vi "ReadTDMSFileFromHBM&Correct.vi"(4 "error in (no error)":errorcluster, 6 "file path":path) -> (0 "sortie d'erreur":errorcluster, 2 "HBMWaveformsOut":waveform(dbl)[](graph))   [LabVIEW 2017]
panel:
  out "Graphe":waveform(dbl)[](graph)
  out "iteraFinal":i32
  out "TabNomFinal":string[](array[string])
  out "ChannelNames 2":string[](array[string])
  out "size(s) 3":i32
  out "WaveformComputational":waveform(dbl)[](graph)
  out "ChannelUnit 2":string[](array[string])
  out "size(s) 2":i32
  out "Unit":string
  out "Name":string
  out "ChannelUnit":string[](array[string])
  out "ChannelNames":string[](array[string])
  out "Waveform Graph 2":waveform(dbl)(graph)
  out "WaveformHardware":waveform(dbl)[](graph)
  out "size(s)":i32
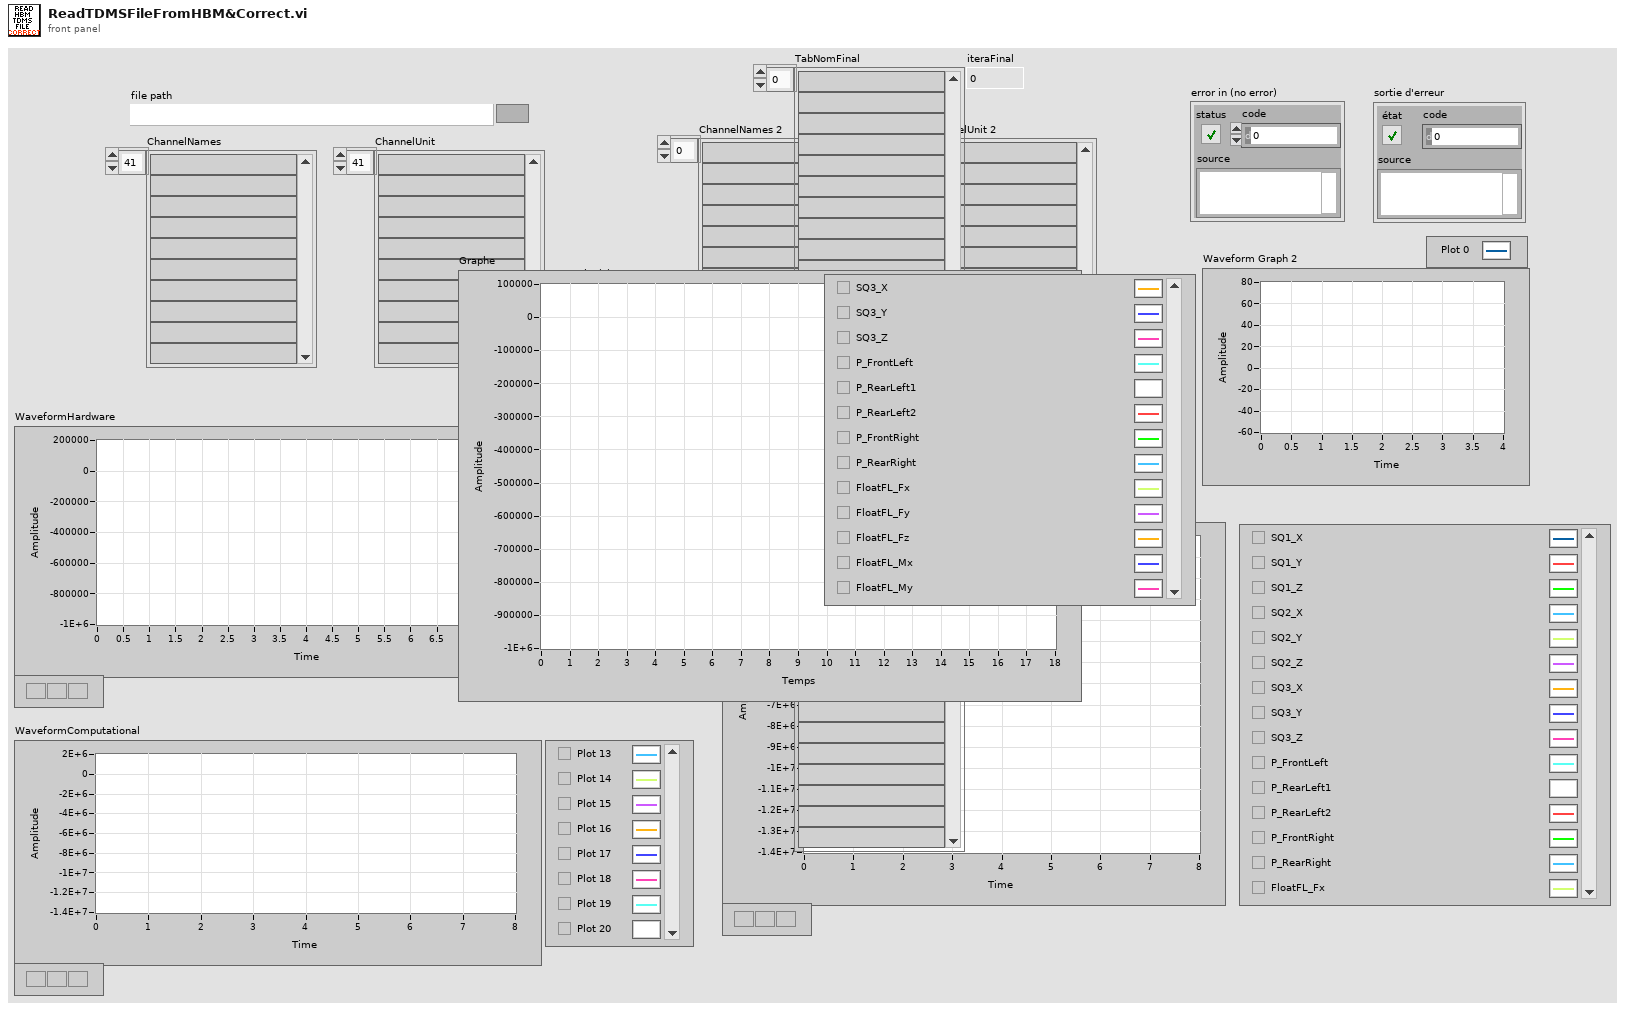
[diagram p1: front panel]
types:
  T1 = enum16{"open", "open or create", "create or replace", "create", "open (read-only)"}
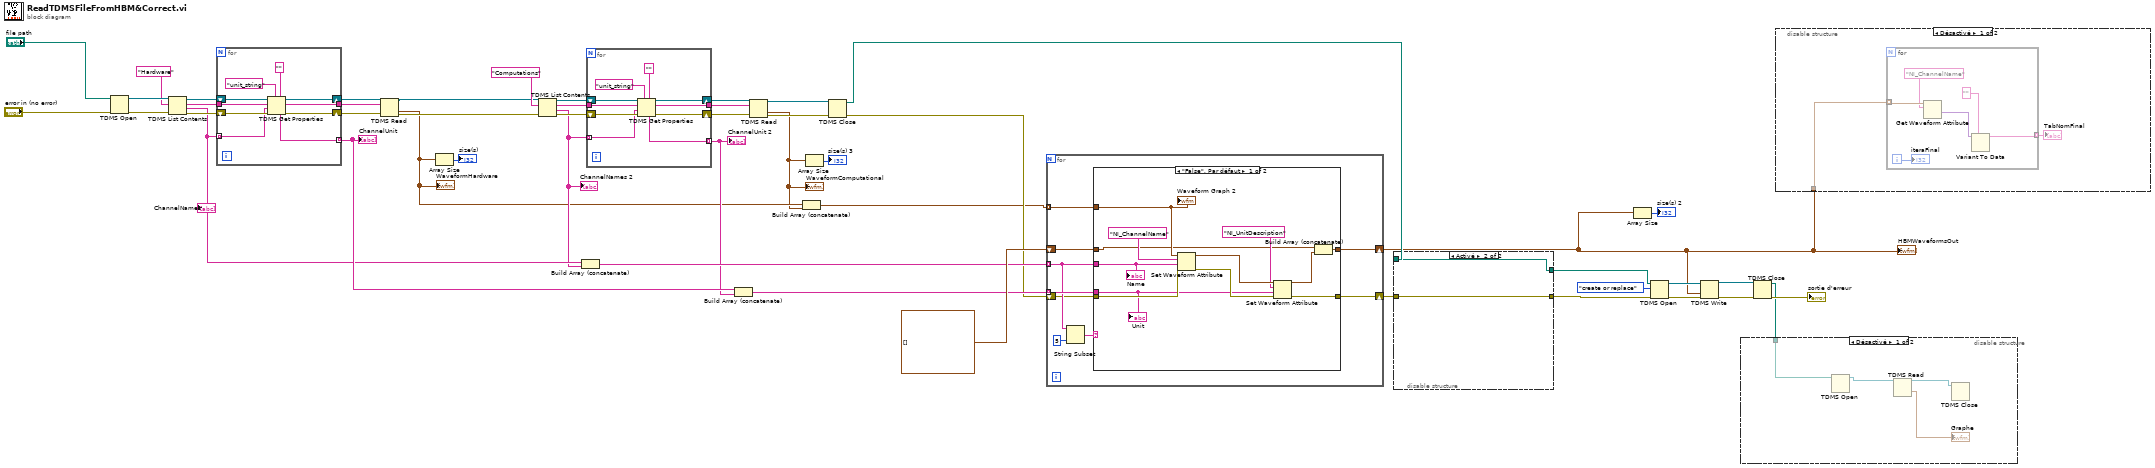
[diagram p0: block diagram]
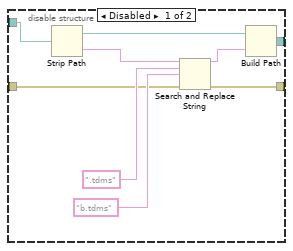
[diagram p2: hidden frame]
diagram:
  n1 = TDMS Open(8:"error in (no error)", 11:"file path") -> (0:w46:errorcluster, 3:w45:refnum<k34>)  [unwired: 5 in]
  n2 = TDMS List Contents(4:w46, 6:"Hardware" ("group name"), 7:w45) -> (0:w43:errorcluster, 1:w18:string[], 2:w41:string, 3:w44:refnum<k34>)
  "ChannelNames" <- w18
  n3 = for {
    tunnel: w41 -> [w54]
    shift-right: [w56] -> w40
    shift-left: w44 -> [w58]
    shift-right: [w55] -> w39
    shift-left: w43 -> [w57]
    tunnel: w18 -> [w51] mode=indexing
    tunnel: [w50] -> w20 mode=indexing
    tunnel: [w49] -> w38
    n4 = TDMS Get Properties(5:"" ("property name"), 7:"unit_string" ("property name"), 8:w57, 9:w51, 10:w54, 11:w58) -> (0:w55:errorcluster, 2:w49:string, 3:w56:refnum<k34>, 4:w50:string)  [unwired: 2 out]
  }
  "ChannelUnit" <- w20
  n5 = TDMS Read(0:w40, 5:w38, 11:w39) -> (4:w24:refnum<k34>, 10:w16:waveform(dbl)[], 15:w25:errorcluster)  [unwired: 5 in, 3 out]
  "WaveformHardware" <- w16
  n6 = Array Size(array=w16) -> (size(s)=→"size(s)":i32)
  n7 = TDMS List Contents(4:w25, 6:"Computations" ("group name"), 7:w24) -> (0:w30:errorcluster, 1:w17:string[], 2:w32:string, 3:w29:refnum<k34>)
  "ChannelNames 2" <- w17
  n8 = Build Array (concatenate)(w18, w17) -> (w23:string[])
  n9 = for {
    tunnel: w32 -> [w64]
    shift-right: [w66] -> w33
    shift-left: w29 -> [w68]
    shift-right: [w65] -> w34
    shift-left: w30 -> [w67]
    tunnel: w17 -> [w61] mode=indexing
    tunnel: [w60] -> w19 mode=indexing
    tunnel: [w59] -> w35
    n10 = TDMS Get Properties(5:"" ("property name"), 7:"unit_string" ("property name"), 8:w67, 9:w61, 10:w64, 11:w68) -> (0:w65:errorcluster, 2:w59:string, 3:w66:refnum<k34>, 4:w60:string)  [unwired: 2 out]
  }
  "ChannelUnit 2" <- w19
  n11 = Build Array (concatenate)(w20, w19) -> (w22:string[])
  n12 = TDMS Read(0:w33, 5:w35, 11:w34) -> (4:w27:refnum<k34>, 10:w15:waveform(dbl)[], 15:w26:errorcluster)  [unwired: 5 in, 3 out]
  "WaveformComputational" <- w15
  n13 = Build Array (concatenate)(w16, w15) -> (w14:waveform(dbl)[])
  n14 = Array Size(array=w15) -> (size(s)=→"size(s) 3":i32)
  n15 = TDMS Close(8:w26, 11:w27) -> (0:w21:errorcluster, 3:w4:path)
  n16 = for {
    tunnel: w14 -> [w77] mode=indexing
    tunnel: w23 -> [w74] mode=indexing
    tunnel: w22 -> [w76] mode=indexing
    shift-right: [w71] -> w2
    shift-left: waveform(dbl)[] [] -> [w70]
    shift-right: [w75] -> w6
    shift-left: w21 -> [w69]
    n17 = String Subset(string=w74, length (rest)=5 ("length (rest)")) -> (substring=w72:string)  [unwired: 1 in]
    n18 = case shown="\"False\", Par défaut" w72 {
      tunnel: w69 -> [w89 w90]
      tunnel: w77 -> [w88 _]
      tunnel: w76 -> [w83 _]
      tunnel: [w82 w90] -> w75
      tunnel: w74 -> [w81 _]
      tunnel: [w79 w91] -> w71
      tunnel: w70 -> [w78 w91]
      frame "False", Default {
        n19 = Set Waveform Attribute(4:w89, 5:w81, 6:"NI_ChannelName" ("name"), 7:w88) -> (0:w87:errorcluster, 3:w86:waveform(dbl))  [unwired: 1 out]
        n20 = Set Waveform Attribute(4:w87, 5:w83, 6:"NI_UnitDescription" ("name"), 7:w86) -> (0:w82:errorcluster, 3:w80:waveform(dbl))  [unwired: 1 out]
        n21 = Build Array (concatenate)(w78, w80) -> (w79:waveform(dbl)[])
        "Waveform Graph 2" <- w88
        "Name" <- w81
        "Unit" <- w83
      }
      frame "Temps" {
      }
    }
  }
  "HBMWaveformsOut" <- w2
  n22 = disable-structure shown="Activé" {
    disable-tunnel: w6 -> [w98 w101]
    disable-tunnel: [w97 w101] -> w5
    disable-tunnel: w4 -> [w96 w102]
    disable-tunnel: [w92 w102] -> w3
    frame Disabled {
      n23 = Strip Path(path=w96) -> (stripped path=w94:path, name=w95:string)
      n24 = Search and Replace String(input string=w95, search string=".tdms" ("sous-chaîne (\"\")"), replace string="b.tdms" ("sous-chaîne (\"\")"), error in=w98) -> (result string=w93:string, error out=w97:errorcluster)  [unwired: 4 in, 2 out]
      n25 = Build Path(base path=w94, name or relative path=w93) -> (appended path=w92:path)
    }
    frame Enabled {
    }
  }
  n26 = Array Size(array=w2) -> (size(s)=→"size(s) 2":i32)
  n27 = TDMS Open(8:w5, 10:T1."create or replace" ("opération (0 : open)"), 11:w3) -> (0:w13:errorcluster, 3:w11:refnum<k34>)  [unwired: 4 in]
  n28 = TDMS Write(0:w11, 9:w2, 11:w13) -> (4:w10:refnum<k34>, 15:w12:errorcluster)  [unwired: 3 in, 2 out]
  n29 = TDMS Close(8:w12, 11:w10) -> (0:→"sortie d'erreur":errorcluster, 3:w1:path)
  n30 = disable-structure shown="Désactivé" {
    disable-tunnel: w1 -> [w106 _]
    frame Disabled {
      n31 = TDMS Open(11:w106) -> (3:w105:refnum<k34>)  [unwired: 6 in, 1 out]
      n32 = TDMS Read(0:w105) -> (4:w104:refnum<k34>, 10:→"Graphe":waveform(dbl)[])  [unwired: 7 in, 4 out]
      n33 = TDMS Close(11:w104) -> ()  [unwired: 1 in, 2 out]
    }
    frame Enabled {
    }
  }
  n34 = disable-structure shown="Désactivé" {
    disable-tunnel: w2 -> [w108 _]
    frame Disabled {
      n35 = for {
        tunnel: w108 -> [w114] mode=indexing
        tunnel: [w110] -> w107 mode=indexing
        i -> [w109]
        n36 = Get Waveform Attribute(6:"NI_ChannelName" ("name"), 7:w114) -> (1:w112:variant)  [unwired: 2 in, 3 out]
        n37 = Variant To Data(type="" ("name"), Variant=w112) -> (data=w110:string)  [unwired: 1 in, 1 out]
        "iteraFinal" <- w109
      }
      "TabNomFinal" <- w107
    }
    frame Enabled {
    }
  }
